vi "polymorphism of arithmetic functions.vi"() -> ()   [LabVIEW 2016]
panel:
  out "Waveform Graph":dbl[][](graph)
  in  "Scale":dbl
  out "Array1 + Array2":dbl[](array[numeric])
  out "Array1* Scale":dbl[](array[numeric])
  out "Array2":dbl[](array[numeric])
  out "Array1":dbl[](array[numeric])
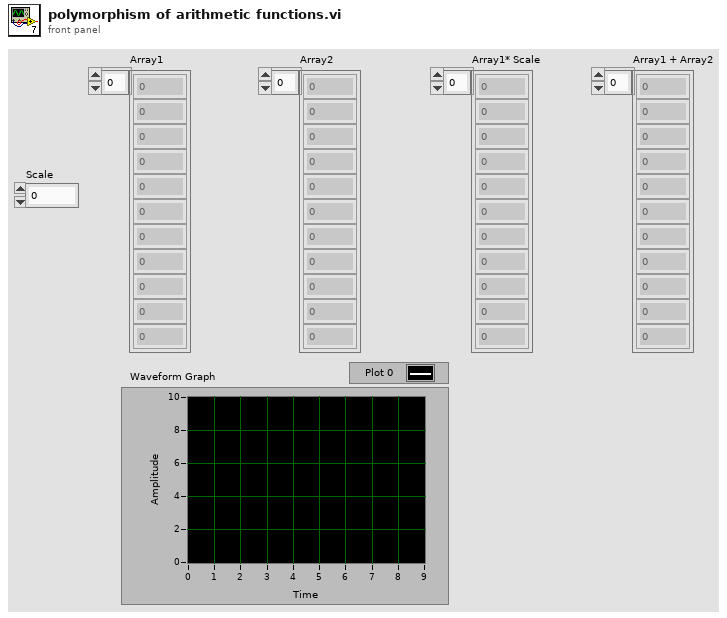
[diagram p1: front panel]
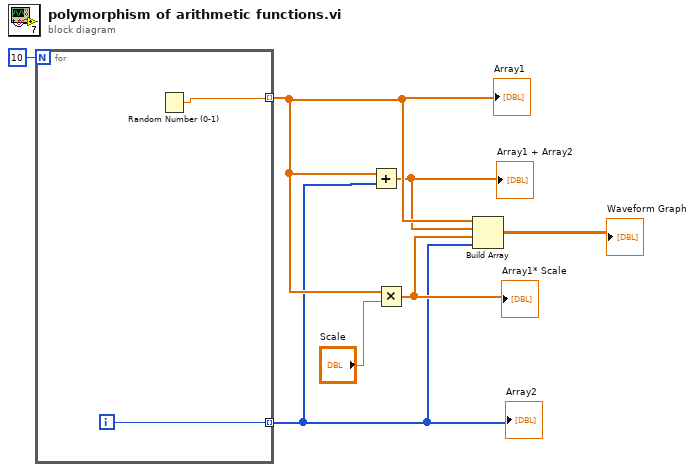
[diagram p0: block diagram]
diagram:
  n1 = for {
    N: 10 -> [_]
    tunnel: [w9] -> w5 mode=indexing
    tunnel: [w8] -> w2 mode=indexing
    i -> [w8]
    n2 = Random Number (0-1)() -> (number: 0 to 1=w9:dbl)
  }
  "Array1" <- w5
  "Array2" <- w2
  n3 = Add(x=w5, y=w2) -> (x+y=w4:dbl[])
  "Array1 + Array2" <- w4
  n4 = Multiply(x=w5, y="Scale") -> (x*y=w3:dbl[])
  "Array1* Scale" <- w3
  n5 = Build Array(w5, w4, w3, w2) -> (→"Waveform Graph":dbl[][])
